vi "poly_recursive_get_cluster_element(s).vi"(7 "delimiter (/)":string="/", 8 "error in (no error)":errorcluster, 9 "field name":string, 11 "Cluster":variant) -> (0 "error out":errorcluster, 1 "Data":variant, 2 "found?":bool, 3 "Cluster out":variant)   [LabVIEW 2015]
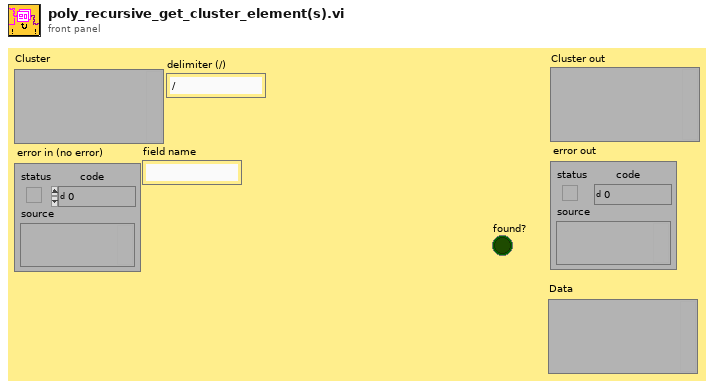
[diagram p1: front panel]
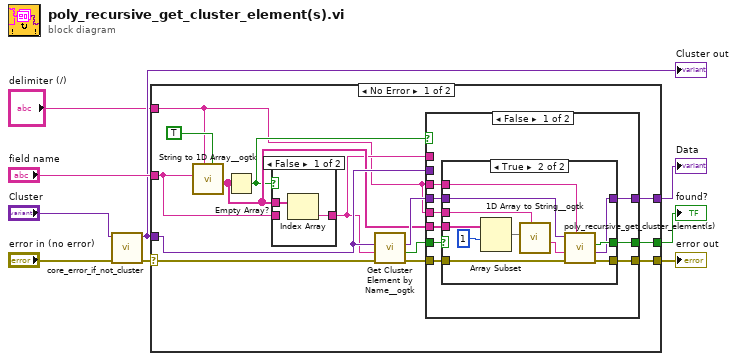
[diagram p0: block diagram]
diagram:
  n1 = call "core_error_if_not_cluster.vi"("Error in"="error in (no error)", "Cluster"="Cluster") -> ("Error out"=w2:errorcluster, "Cluster duplicate"=w3:variant)  [unwired: 8 in]
  "Cluster out" <- w3
  n2 = case shown="No Error" w2 {
    selector: w2 -> [w15 w53]
    tunnel: w3 -> [w22 _]
    tunnel: [w16 w53] -> w9
    tunnel: "field name" -> [w14 _]
    tunnel: [w20 _] -> w8
    tunnel: [w19 _] -> w6
    tunnel: "delimiter (/)" -> [w10 _]
    frame No Error {
      n3 = call <userlib>:"String to 1D Array__ogtk.vi"("ignore duplicate delimiters? (F=No)"=TRUE, "delimiter (Tab)"=w10, "string"=w14) -> ("Array of Strings"=w13:string[])  [unwired: 8 in]
      n4 = Empty Array?(array=w13) -> (empty?=w11:bool)
      n5 = case shown="False" w11 {
        tunnel: w14 -> [_ w26]
        tunnel: w13 -> [w25 _]
        tunnel: [w24 w26] -> w12
        frame False {
          n6 = Index Array(array=w25) -> (element=w24:string)  [unwired: 1 in]
        }
        frame True {
        }
      }
      n7 = call <userlib>:"Get Cluster Element by Name__ogtk.vi"("error in (no error)"=w15, "Element Name"=w12, "Cluster"=w22) -> ("error out"=w17:errorcluster, "found?"=w18:bool, "VElement"=w21:variant)  [unwired: 6 in]
      n8 = case shown="False" w11 {
        tunnel: w12 -> [_ _]
        tunnel: w22 -> [_ _]
        tunnel: w10 -> [w35 _]
        tunnel: w21 -> [w34 w52]
        tunnel: w13 -> [w33 _]
        tunnel: [w32 w51] -> w20
        tunnel: [w31 w52] -> w19
        tunnel: w18 -> [w30 w51]
        tunnel: w17 -> [w29 w50]
        tunnel: [w28 w50] -> w16
        tunnel: w10 -> [w27 _]
        frame False {
          n9 = case shown="True" w30 {
            selector: w30 -> [w38 _]
            tunnel: w35 -> [_ w49]
            tunnel: w34 -> [w37 w47]
            tunnel: w33 -> [_ w45]
            tunnel: [w38 w43] -> w32
            tunnel: [w37 w42] -> w31
            tunnel: w29 -> [w36 w41]
            tunnel: [w36 w40] -> w28
            tunnel: w27 -> [_ w39]
            frame False {
            }
            frame True {
              n10 = Array Subset(array=w45, index=1) -> (w44:string[])  [unwired: 1 in]
              n11 = call <userlib>:"1D Array to String__ogtk.vi"("delimiter (Tab)"=w49, "Array of Strings"=w44) -> ("delimited string"=w48:string)  [unwired: 9 in]
              n12 = call "poly_recursive_get_cluster_element(s).vi"("delimiter (/)"=w39, "error in (no error)"=w41, "field name"=w48, "Cluster"=w47) -> ("error out"=w40:errorcluster, "Data"=w42:variant, "found?"=w43:bool)  [unwired: 4 in, 1 out]
            }
          }
        }
        frame True {
        }
      }
    }
    frame Error {
    }
  }
  "Data" <- w6
  "error out" <- w9
  "found?" <- w8
